vi "Histogram Main.vi"() -> ()   [LabVIEW 2014]
uses:
  Consumer Message.ctl
  <vilib>/Utility/file.llb/Write To Spreadsheet File (DBL).vi
  <vilib>/ErrorRing/Error Ring.xnode
panel:
  in  "signal":u16(ring) items=["uniform white", "uniform+uniform", "Gaussian white", "sine", "square"]
  in  "Snapshot":bool
  out "Histogram":cluster{"histogram":dbl[], "x axis":dbl[]}(graph)
  in  "bins":i32=20
  out "Consumer Shutdown?":bool
  out "Backlog":u8(slide) scale=0.0..100.0
  in  "Stop":bool
  # "Number of enqueued messages waiting to be processed"
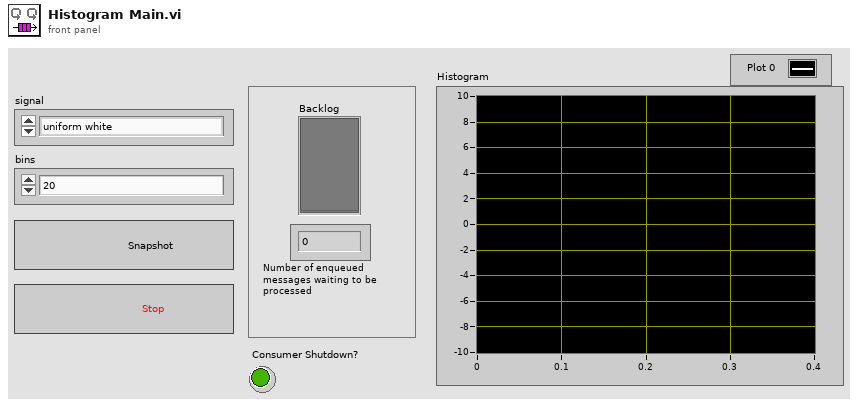
[diagram p1: front panel]
types:
  T1 = typedef "Consumer Message.ctl" = cluster{"Consumer State":string, "Boolean Data":bool, "Numeric Data":i32, "Signal":dbl[], "Error":errorcluster}
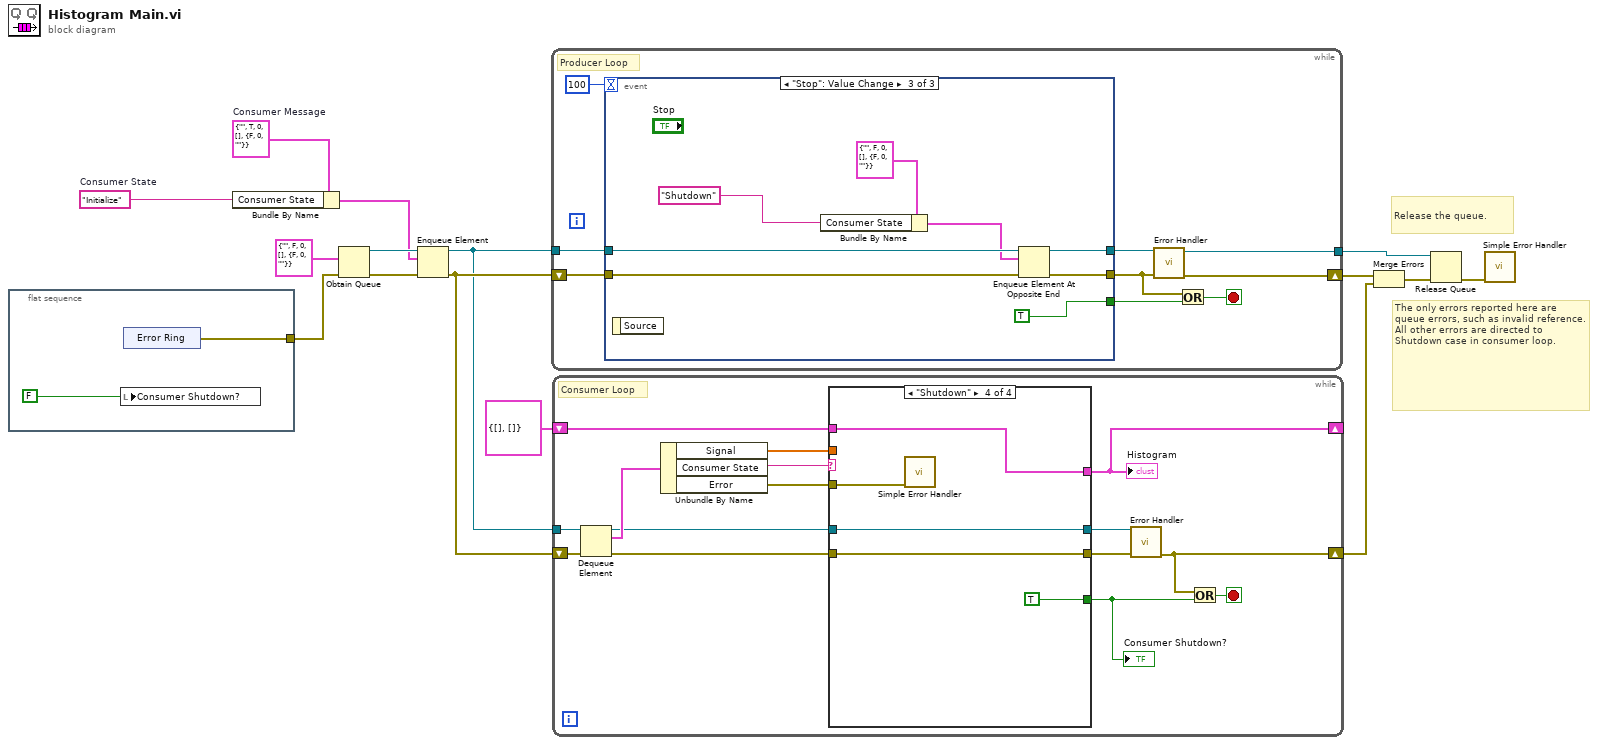
[diagram p0: block diagram]
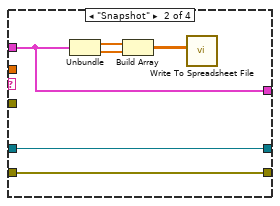
[diagram p3: hidden frame]
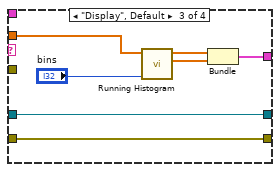
[diagram p4: hidden frame]
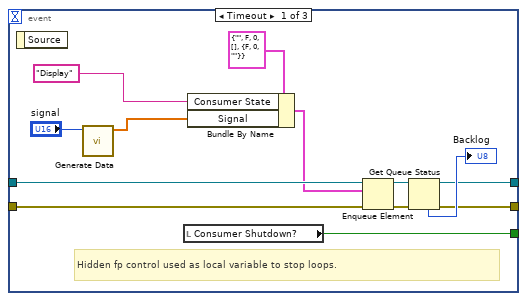
[diagram p5: hidden frame]
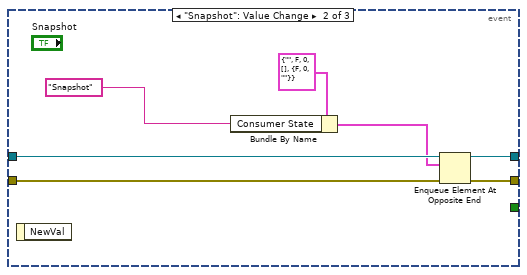
[diagram p6: hidden frame]
diagram:
  w4 = T1 {"Consumer State"="", "Boolean Data"=TRUE, "Numeric Data"=0, "Signal"=[], "Error"={"status"=FALSE, "code"=0, "source"=""}}  # Consumer Message
  w8 = "Initialize"  # Consumer State
  # "Release the queue."
  # "The only errors reported here are queue errors, such as invalid reference.  All other errors are directed to Shutdown case in consumer loop."
  n1 = flat-sequence {
    tunnel: [w16] -> w10
    frame #0 {
      n2 = local write "Consumer Shutdown?"(FALSE ("Stop Loops (local)")) -> ()
      n3 = xnode "Error Ring"() -> ("error out"=w16:errorcluster)
    }
  }
  n4 = Bundle By Name(cluster=w4, "Consumer State"=w8) -> (w9:T1)
  n5 = Obtain Queue(element data type=T1 {"Consumer State"="", "Boolean Data"=FALSE, "Numeric Data"=0, "Signal"=[], "Error"={"status"=FALSE, "code"=0, "source"=""}}, error in (no error)=w10) -> (queue out=w12:refnum<queue>, error out=w15:errorcluster)  [unwired: 3 in, 1 out]
  n6 = Enqueue Element(queue=w12, element=w9, error in (no error)=w15) -> (queue out=w11:refnum<queue>, error out=w13:errorcluster)  [unwired: 1 in, 1 out]
  n7 = while {
    tunnel: w11 -> [w27]
    shift-right: [w20] -> w7
    shift-left: w13 -> [w26]
    tunnel: [w19] -> w1
    stop <- w22 stop-if-true
    # "Producer Loop"
    n8 = event shown="[2] \"Stop\": Value Change" {
      selector: _ -> [_ _ _]
      dyn-events: _ -> [_ _ _]
      timeout: 100 -> [_ _ _]
      tunnel: w27 -> [w38 w46 w55]
      tunnel: w26 -> [w34 w45 w53]
      tunnel: [w37 w47 w52] -> w21
      tunnel: [w40 _ TRUE] -> w23
      tunnel: [w36 w42 w51] -> w25
      event Timeout {
        # "Hidden fp control used as local variable to stop loops."
        n9 = event-data() -> ()  [unwired: 1 in, 1 out]
        n10 = call "Generate Data.vi"("signal"="signal") -> ("Y"=w30:dbl[])  [unwired: 9 in, 1 out]
        n11 = local read "Consumer Shutdown?"() -> (w40:bool)
        n12 = Bundle By Name(cluster=T1 {"Consumer State"="", "Boolean Data"=FALSE, "Numeric Data"=0, "Signal"=[], "Error"={"status"=FALSE, "code"=0, "source"=""}}, "Consumer State"="Display", "Signal"=w30) -> (w31:T1)
        n13 = Enqueue Element(queue=w38, element=w31, error in (no error)=w34) -> (queue out=w35:refnum<queue>, error out=w33:errorcluster)  [unwired: 1 in, 1 out]
        n14 = Get Queue Status(queue=w35, error in (no error)=w33) -> (queue out=w36:refnum<queue>, error out=w37:errorcluster, # elements in queue=→"Backlog":i32)  [unwired: 1 in, 5 out]
      }
      event "Snapshot": Value Change {
        n15 = event-data() -> ()  [unwired: 1 in, 1 out]
        n16 = Bundle By Name(cluster=T1 {"Consumer State"="", "Boolean Data"=FALSE, "Numeric Data"=0, "Signal"=[], "Error"={"status"=FALSE, "code"=0, "source"=""}}, "Consumer State"="Snapshot" ("String Data")) -> (w43:T1)
        n17 = Enqueue Element At Opposite End(queue=w46, element=w43, error in (no error)=w45) -> (queue out=w42:refnum<queue>, error out=w47:errorcluster)  [unwired: 1 in, 1 out]
      }
      event "Stop": Value Change {
        n18 = event-data() -> ()  [unwired: 1 in, 1 out]
        n19 = Bundle By Name(cluster=T1 {"Consumer State"="", "Boolean Data"=FALSE, "Numeric Data"=0, "Signal"=[], "Error"={"status"=FALSE, "code"=0, "source"=""}}, "Consumer State"="Shutdown") -> (w48:T1)
        n20 = Enqueue Element At Opposite End(queue=w55, element=w48, error in (no error)=w53) -> (queue out=w51:refnum<queue>, error out=w52:errorcluster)  [unwired: 1 in, 1 out]
      }
    }
    n21 = call "Error Handler.vi"("error in"=w21, "queue in"=w25) -> ("error out"=w20:errorcluster, "queue out"=w19:refnum<queue>)  [unwired: 8 in]
    n22 = Or(x=w21, y=w23) -> (x .or. y?=w22:bool)
  }
  n23 = while {
    tunnel: w11 -> [w70]
    shift-right: [w61] -> w6
    shift-left: w13 -> [w69]
    shift-right: [w58] -> _
    shift-left: cluster{"histogram":dbl[], "x axis":dbl[]} {"histogram"=[], "x axis"=[]} -> [w57]
    stop <- w62 stop-if-true
    # "Consumer Loop"
    n24 = Dequeue Element(queue=w70, error in (no error)=w69) -> (queue out=w60:refnum<queue>, element=w68:T1, error out=w59:errorcluster)  [unwired: 1 in, 1 out]
    n25 = Unbundle By Name(w68) -> ("Signal"=w56:dbl[], "Consumer State"=w67:string, "Error"=w64:errorcluster)
    n26 = case shown="\"Shutdown\"" w67 {
      tunnel: [_ _ _ TRUE] -> w63
      tunnel: w59 -> [w72 w78 w85 w87]
      tunnel: [w72 w78 w85 w87] -> w66
      tunnel: w60 -> [w73 w79 w86 w89]
      tunnel: [w73 w79 w86 w89] -> w65
      tunnel: w64 -> [_ _ _ w90]
      tunnel: [w71 w74 w81 w88] -> w58
      tunnel: w57 -> [w71 w74 _ w88]
      tunnel: w56 -> [_ _ w80 _]
      frame "Initialize" {
      }
      frame "Snapshot" {
        n27 = Unbundle(w74) -> ("histogram"=w77:dbl[], "x axis"=w76:dbl[])
        n28 = Build Array(w77, w76) -> (w75:dbl[][])
        n29 = call-poly <vilib>:"Write To Spreadsheet File.vi"("2D data"=w75) -> ()  [unwired: 7 in, 1 out]
      }
      frame "Display", Default {
        n30 = call "Running Histogram.vi"("bins"="bins", "input data"=w80) -> ("x axis"=w82:dbl[], "histogram"=w83:dbl[])  [unwired: 6 in, 2 out]
        n31 = Bundle("histogram"=w83, "x axis"=w82) -> (w81:cluster{"histogram":dbl[], "x axis":dbl[]})  [unwired: 1 in]
      }
      frame "Shutdown" {
        n32 = call <vilib>:"Simple Error Handler.vi"("error in (no error)"=w90) -> ()  [unwired: 4 in, 5 out]
      }
    }
    "Consumer Shutdown?" <- w63
    "Histogram" <- w58
    n33 = call "Error Handler.vi"("error in"=w66, "queue in"=w65) -> ("error out"=w61:errorcluster)  [unwired: 8 in, 1 out]
    n34 = Or(x=w61, y=w63) -> (x .or. y?=w62:bool)
  }
  n35 = Merge Errors(w7, w6) -> (w3:errorcluster)
  n36 = Release Queue(queue=w1, error in (no error)=w3) -> (error out=w2:errorcluster)  [unwired: 1 in, 2 out]
  n37 = call <vilib>:"Simple Error Handler.vi"("error in (no error)"=w2) -> ()  [unwired: 4 in, 5 out]
